vi "Data From Memory.vi"() -> (3 "DSM Message":string)   [LabVIEW 2014]
uses:
  Custom Pallet Controls/Forward.ctl
panel:
  in  "Address LSBL":u16
  in  "Address LSBH":u16
  in  "Address MSBL":u16
  in  "Address MSBH":u16
  in  "Number of Bytes (up to 16)":u16
  out "Description":string="Set Currents"
  in  "Complete":T1
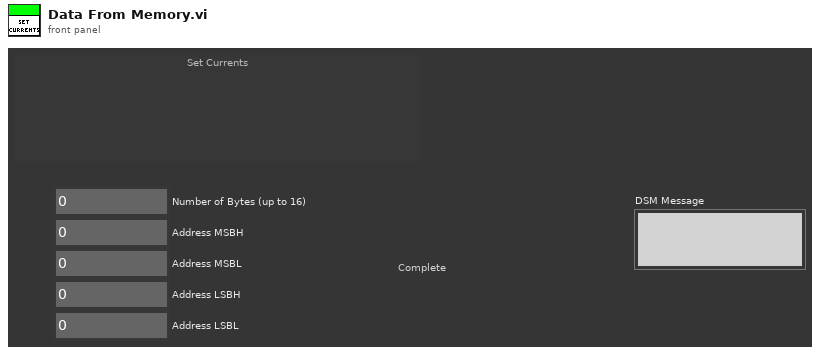
[diagram p1: front panel]
types:
  T1 = typedef "Forward.ctl" = bool
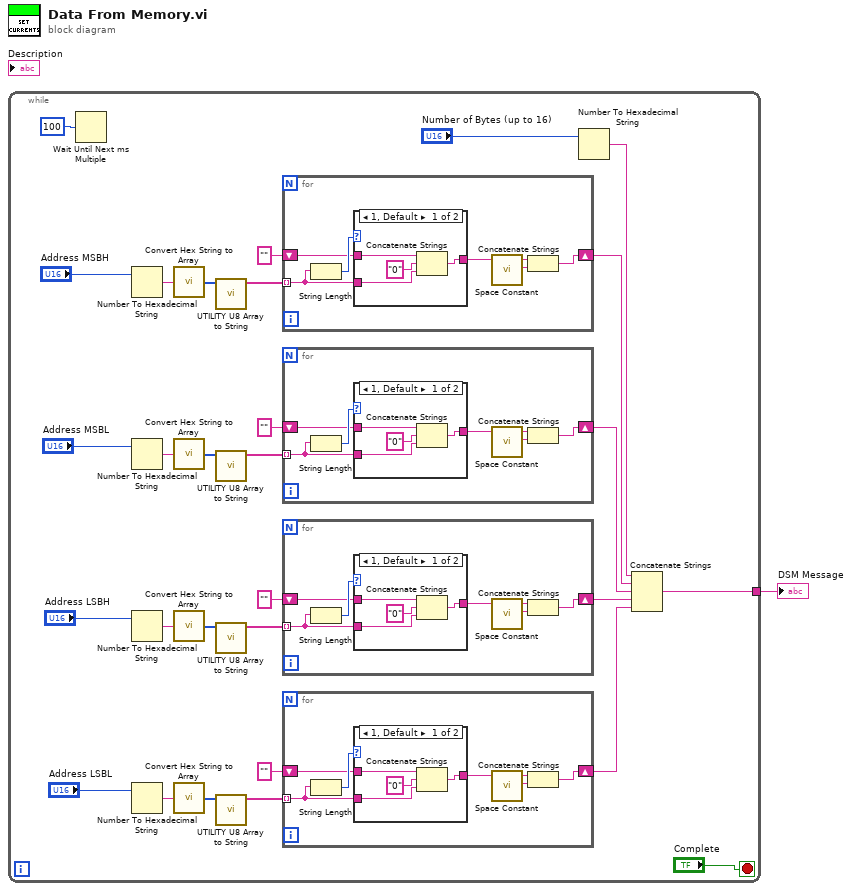
[diagram p0: block diagram]
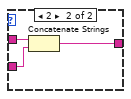
[diagram p2: hidden frame]
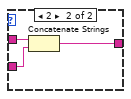
[diagram p3: hidden frame]
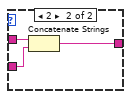
[diagram p4: hidden frame]
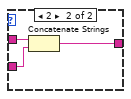
[diagram p5: hidden frame]
diagram:
  n1 = while {
    tunnel: [w18] -> w1
    stop <- "Complete" stop-if-true
    n2 = Wait Until Next ms Multiple(millisecond multiple=u32 100) -> ()  [unwired: 1 out]
    n3 = Number To Hexadecimal String(2:"Address MSBH") -> (0:w22:string)  [unwired: 1 in]
    n4 = Number To Hexadecimal String(2:"Address MSBL") -> (0:w24:string)  [unwired: 1 in]
    n5 = Number To Hexadecimal String(2:"Address LSBH") -> (0:w26:string)  [unwired: 1 in]
    n6 = Number To Hexadecimal String(2:"Address LSBL") -> (0:w12:string)  [unwired: 1 in]
    n7 = call "Convert Hex String to Array.vi"("Hex String In"=w22) -> ("Hex Array Out"=w9:u8[])  [unwired: 14 in]
    n8 = call "Convert Hex String to Array.vi"("Hex String In"=w24) -> ("Hex Array Out"=w7:u8[])  [unwired: 14 in]
    n9 = call "Convert Hex String to Array.vi"("Hex String In"=w26) -> ("Hex Array Out"=w5:u8[])  [unwired: 14 in]
    n10 = call "Convert Hex String to Array.vi"("Hex String In"=w12) -> ("Hex Array Out"=w3:u8[])  [unwired: 14 in]
    n11 = call "UTILITY U8 Array to String.vi"("Hex Array Out"=w9) -> ("Array"=w8:string[])  [unwired: 10 in]
    n12 = call "UTILITY U8 Array to String.vi"("Hex Array Out"=w7) -> ("Array"=w6:string[])  [unwired: 10 in]
    n13 = call "UTILITY U8 Array to String.vi"("Hex Array Out"=w5) -> ("Array"=w4:string[])  [unwired: 10 in]
    n14 = call "UTILITY U8 Array to String.vi"("Hex Array Out"=w3) -> ("Array"=w2:string[])  [unwired: 10 in]
    n15 = for {
      tunnel: w8 -> [w73] mode=indexing
      shift-right: [w70] -> w21
      shift-left: "" -> [w74]
      n16 = String Length(string=w73) -> (length=w75:i32)
      n17 = case shown="1, Default" w75 {
        tunnel: w74 -> [w79 w82]
        tunnel: [w76 w81] -> w71
        tunnel: w73 -> [w77 w80]
        frame 1, Default {
          n18 = Concatenate Strings(w79, "0" ("string"), w77) -> (w76:string)
        }
        frame 2 {
          n19 = Concatenate Strings(w82, w80) -> (w81:string)
        }
      }
      n20 = call <vilib>:"Space Constant.vi"() -> ("String"=w72:string)
      n21 = Concatenate Strings(w71, w72) -> (w70:string)
    }
    n22 = for {
      tunnel: w6 -> [w60] mode=indexing
      shift-right: [w57] -> w20
      shift-left: "" -> [w61]
      n23 = String Length(string=w60) -> (length=w62:i32)
      n24 = case shown="1, Default" w62 {
        tunnel: w61 -> [w66 w69]
        tunnel: [w63 w68] -> w58
        tunnel: w60 -> [w64 w67]
        frame 1, Default {
          n25 = Concatenate Strings(w66, "0" ("string"), w64) -> (w63:string)
        }
        frame 2 {
          n26 = Concatenate Strings(w69, w67) -> (w68:string)
        }
      }
      n27 = call <vilib>:"Space Constant.vi"() -> ("String"=w59:string)
      n28 = Concatenate Strings(w58, w59) -> (w57:string)
    }
    n29 = for {
      tunnel: w4 -> [w47] mode=indexing
      shift-right: [w44] -> w19
      shift-left: "" -> [w48]
      n30 = String Length(string=w47) -> (length=w49:i32)
      n31 = case shown="1, Default" w49 {
        tunnel: w48 -> [w53 w56]
        tunnel: [w50 w55] -> w45
        tunnel: w47 -> [w51 w54]
        frame 1, Default {
          n32 = Concatenate Strings(w53, "0" ("string"), w51) -> (w50:string)
        }
        frame 2 {
          n33 = Concatenate Strings(w56, w54) -> (w55:string)
        }
      }
      n34 = call <vilib>:"Space Constant.vi"() -> ("String"=w46:string)
      n35 = Concatenate Strings(w45, w46) -> (w44:string)
    }
    n36 = for {
      tunnel: w2 -> [w34] mode=indexing
      shift-right: [w31] -> w10
      shift-left: "" -> [w35]
      n37 = String Length(string=w34) -> (length=w36:i32)
      n38 = case shown="1, Default" w36 {
        tunnel: w35 -> [w40 w43]
        tunnel: [w37 w42] -> w32
        tunnel: w34 -> [w38 w41]
        frame 1, Default {
          n39 = Concatenate Strings(w40, "0" ("string"), w38) -> (w37:string)
        }
        frame 2 {
          n40 = Concatenate Strings(w43, w41) -> (w42:string)
        }
      }
      n41 = call <vilib>:"Space Constant.vi"() -> ("String"=w33:string)
      n42 = Concatenate Strings(w32, w33) -> (w31:string)
    }
    n43 = Number To Hexadecimal String(2:"Number of Bytes (up to 16)") -> (0:w14:string)  [unwired: 1 in]
    n44 = Concatenate Strings(w14, w21, w20, w19, w10) -> (w18:string)
  }
  "DSM Message" <- w1
